vi "IntakeStateMachine.vi"(6 "IntakeCurrent":dbl, 8 "SlowButton":bool, 9 "FastButton":bool, 10 "Joystick":dbl(slide) scale=-1.0..1.0, 11 "Cluster":T1={"OutakeSpeed"=0.4, "OutakeSpeed Fast"=1.0, "Intake Sens"=1.2, "OutakeSens"=0.7} {"OutakeSpeed Fast" format="%#_13g"; "OutakeSpeed" format="%#_13g"}) -> (2 "Left Intake":dbl format="%#_13g", 3 "Right Intake":dbl)   [LabVIEW 2017]
uses:
  Implementation/IntakeStates.ctl
panel:
  out "Waveform Chart":dbl(graph)
  in  "DislodgingLeftSpeed":dbl=-0.2 format="%#_13g"
  in  "DislodgingRightSpeed":dbl=-1.0 format="%#_13g"
  in  "Time Limit":u32=300
  in  "Max Curretnt":dbl=55.0
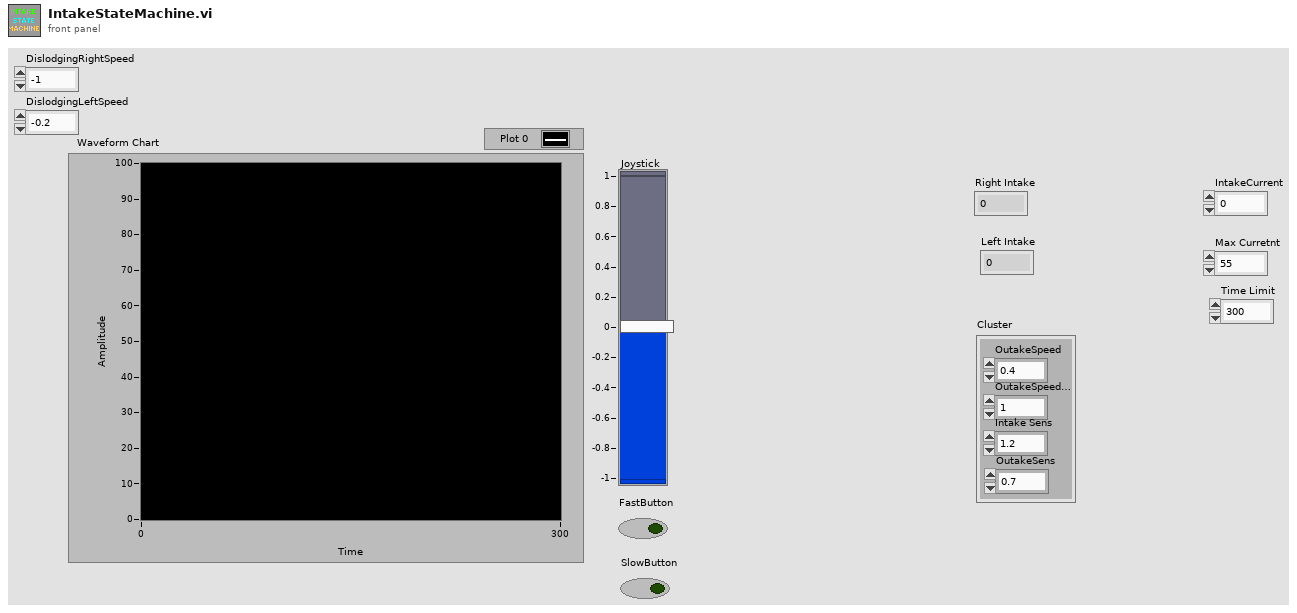
[diagram p1: front panel]
types:
  T1 = cluster{"OutakeSpeed":dbl, "OutakeSpeed Fast":dbl, "Intake Sens":dbl, "OutakeSens":dbl}
  T2 = typedef "IntakeStates.ctl" = enum16{"Intake Manual", "Outtake Manual", "Fast Auto Outake", "Slow Auto Outake", "Dislodging"}
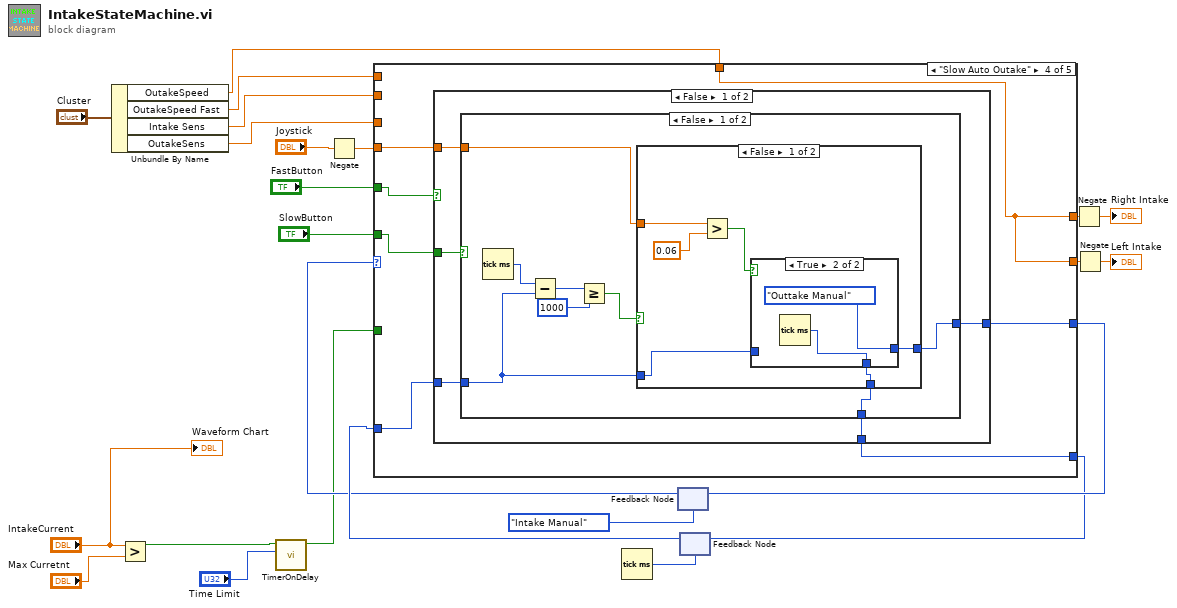
[diagram p0: block diagram]
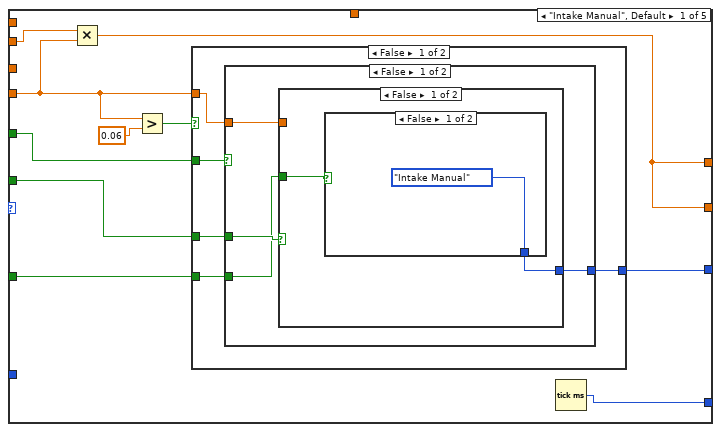
[diagram p2: hidden frame]
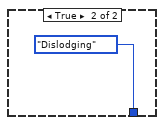
[diagram p3: hidden frame]
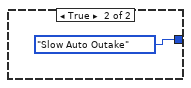
[diagram p4: hidden frame]
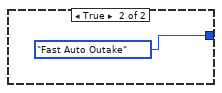
[diagram p5: hidden frame]
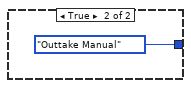
[diagram p6: hidden frame]
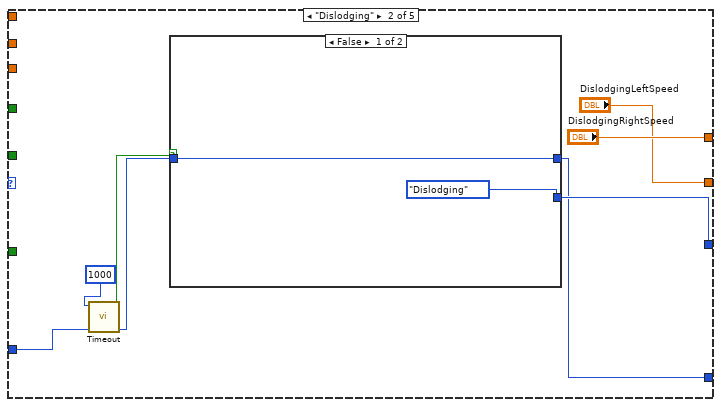
[diagram p7: hidden frame]
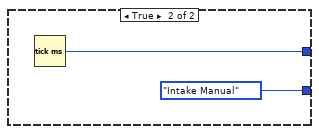
[diagram p8: hidden frame]
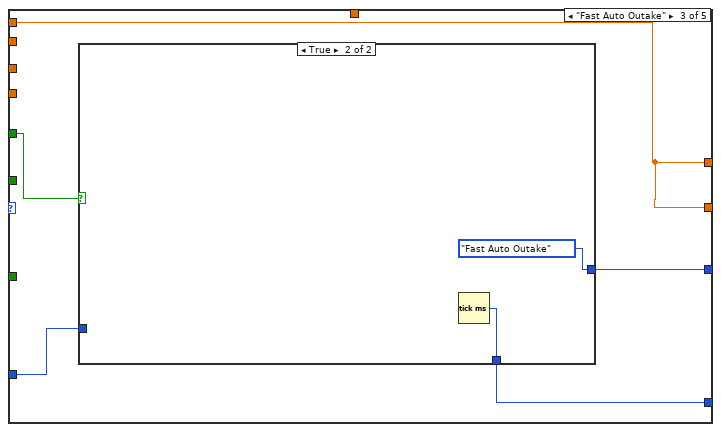
[diagram p9: hidden frame]
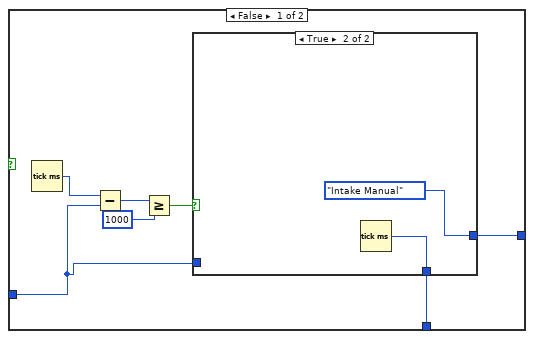
[diagram p10: hidden frame]
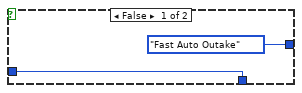
[diagram p11: hidden frame]
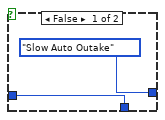
[diagram p12: hidden frame]
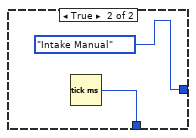
[diagram p13: hidden frame]
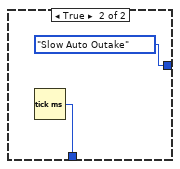
[diagram p14: hidden frame]
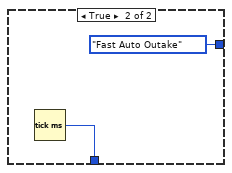
[diagram p15: hidden frame]
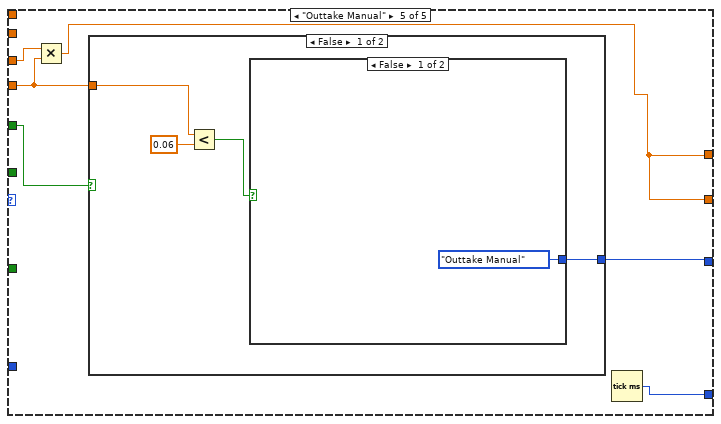
[diagram p16: hidden frame]
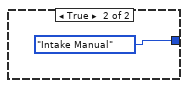
[diagram p17: hidden frame]
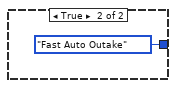
[diagram p18: hidden frame]
diagram:
  n1 = Unbundle By Name("Cluster") -> ("OutakeSpeed"=w14:dbl, "OutakeSpeed Fast"=w15:dbl, "Intake Sens"=w12:dbl, "OutakeSens"=w13:dbl)
  n2 = Greater?(x="IntakeCurrent", y="Max Curretnt") -> (0:w4:bool)
  n3 = call "TimerOnDelay.vi"("Time Limit"="Time Limit", "Input"=w4) -> ("Output"=w2:bool)  [unwired: 9 in]
  n4 = Negate(x="Joystick") -> (-x=w9:dbl)
  n5 = Tick Count (ms)() -> (millisecond timer value=w20:u32)
  n6 = feedback #1(IntakeStates."Intake Manual" ("States")) -> (w11:T2)
  n7 = feedback #2(w20) -> (w19:u32)
  n8 = case shown="\"Slow Auto Outake\"" w11 {
    tunnel: [w26 "DislodgingRightSpeed" w63 w81 w117] -> w17
    tunnel: [w32 w53 w65 w86 w120] -> w23
    tunnel: w9 -> [w28 _ _ w82 w118]
    tunnel: "FastButton" -> [w31 _ w67 w83 w121]
    tunnel: "SlowButton" -> [w30 _ _ w84 _]
    tunnel: w14 -> [_ _ _ w81 _]
    tunnel: w19 -> [_ w56 w64 w85 _]
    tunnel: [w29 w52 w66 w87 w122] -> w18
    tunnel: w15 -> [_ _ w63 _ _]
    tunnel: w13 -> [_ _ _ _ w119]
    tunnel: w12 -> [w27 _ _ _ _]
    tunnel: [w26 "DislodgingLeftSpeed" w63 w81 w117] -> w6
    tunnel: w2 -> [w25 _ _ _ _]
    frame "Intake Manual", Default {
      n9 = Multiply(x=w27, y=w28) -> (x*y=w26:dbl)
      n10 = Greater?(x=w28, y=0.06) -> (0:w33:bool)
      n11 = case shown="False" w33 {
        tunnel: [w38 IntakeStates."Outtake Manual" ("States")] -> w32
        tunnel: w28 -> [w36 _]
        tunnel: w31 -> [w39 _]
        tunnel: w30 -> [w37 _]
        tunnel: w25 -> [w35 _]
        frame False {
          n12 = case shown="False" w39 {
            tunnel: [w42 IntakeStates."Fast Auto Outake" ("States")] -> w38
            tunnel: w37 -> [w43 _]
            tunnel: w36 -> [w41 _]
            tunnel: w35 -> [w40 _]
            frame False {
              n13 = case shown="False" w43 {
                tunnel: [w44 IntakeStates."Slow Auto Outake" ("States")] -> w42
                tunnel: w41 -> [_ _]
                tunnel: w40 -> [w45 _]
                frame False {
                  n14 = case shown="False" w45 {
                    tunnel: [IntakeStates."Intake Manual" ("States") IntakeStates."Dislodging" ("States")] -> w44
                    frame False {
                    }
                    frame True {
                    }
                  }
                }
                frame True {
                }
              }
            }
            frame True {
            }
          }
        }
        frame True {
        }
      }
      n15 = Tick Count (ms)() -> (millisecond timer value=w29:u32)
    }
    frame "Dislodging" {
      n16 = call "Timeout.vi"("Start Time In"=w56, "Time Limit (ms)"=u32 1000) -> ("Start Time Out"=w51:u32, "Timeout"=w54:bool)  [unwired: 8 in]
      n17 = case shown="False" w54 {
        tunnel: [IntakeStates."Dislodging" ("States") IntakeStates."Intake Manual" ("States")] -> w53
        tunnel: [w59 w61] -> w52
        tunnel: w51 -> [w59 _]
        frame False {
        }
        frame True {
          n18 = Tick Count (ms)() -> (millisecond timer value=w61:u32)
        }
      }
    }
    frame "Fast Auto Outake" {
      n19 = case shown="True" w67 {
        tunnel: [w69 w80] -> w66
        tunnel: [w70 IntakeStates."Fast Auto Outake" ("States")] -> w65
        tunnel: w64 -> [w68 _]
        frame False {
          n20 = Tick Count (ms)() -> (millisecond timer value=w74:u32)
          n21 = Subtract(x=w74, y=w68) -> (x-y=w73:u32)
          n22 = Greater Or Equal?(x=w73, y=u32 1000) -> (x >= y?=w71:bool)
          n23 = case shown="True" w71 {
            tunnel: [IntakeStates."Fast Auto Outake" ("States") IntakeStates."Intake Manual" ("States")] -> w70
            tunnel: [w75 w77] -> w69
            tunnel: w68 -> [w75 _]
            frame False {
            }
            frame True {
              n24 = Tick Count (ms)() -> (millisecond timer value=w77:u32)
            }
          }
        }
        frame True {
          n25 = Tick Count (ms)() -> (millisecond timer value=w80:u32)
        }
      }
    }
    frame "Slow Auto Outake" {
      n26 = case shown="False" w83 {
        tunnel: [w92 w115] -> w87
        tunnel: [w91 IntakeStates."Fast Auto Outake" ("States")] -> w86
        tunnel: w85 -> [w90 _]
        tunnel: w84 -> [w89 _]
        tunnel: w82 -> [w88 _]
        frame False {
          n27 = case shown="False" w89 {
            tunnel: [w95 w114] -> w92
            tunnel: [w96 IntakeStates."Slow Auto Outake" ("States")] -> w91
            tunnel: w90 -> [w94 _]
            tunnel: w88 -> [w93 _]
            frame False {
              n28 = Tick Count (ms)() -> (millisecond timer value=w100:u32)
              n29 = Subtract(x=w100, y=w94) -> (x-y=w99:u32)
              n30 = Greater Or Equal?(x=w99, y=u32 1000) -> (x >= y?=w97:bool)
              n31 = case shown="False" w97 {
                tunnel: [w106 IntakeStates."Intake Manual" ("States")] -> w96
                tunnel: [w101 w111] -> w95
                tunnel: w94 -> [w103 _]
                tunnel: w93 -> [w104 _]
                frame False {
                  n32 = Greater?(x=w104, y=0.06) -> (0:w102:bool)
                  n33 = case shown="True" w102 {
                    tunnel: [IntakeStates."Slow Auto Outake" ("States") IntakeStates."Outtake Manual" ("States")] -> w106
                    tunnel: w103 -> [w107 _]
                    tunnel: [w107 w109] -> w101
                    frame False {
                    }
                    frame True {
                      n34 = Tick Count (ms)() -> (millisecond timer value=w109:u32)
                    }
                  }
                }
                frame True {
                  n35 = Tick Count (ms)() -> (millisecond timer value=w111:u32)
                }
              }
            }
            frame True {
              n36 = Tick Count (ms)() -> (millisecond timer value=w114:u32)
            }
          }
        }
        frame True {
          n37 = Tick Count (ms)() -> (millisecond timer value=w115:u32)
        }
      }
    }
    frame "Outtake Manual" {
      n38 = Multiply(x=w119, y=w118) -> (x*y=w117:dbl)
      n39 = case shown="False" w121 {
        tunnel: [w124 IntakeStates."Fast Auto Outake" ("States")] -> w120
        tunnel: w118 -> [w126 _]
        frame False {
          n40 = Less?(x=w126, y=0.06) -> (x < y?=w123:bool)
          n41 = case shown="False" w123 {
            tunnel: [IntakeStates."Outtake Manual" ("States") IntakeStates."Intake Manual" ("States")] -> w124
            frame False {
            }
            frame True {
            }
          }
        }
        frame True {
        }
      }
      n42 = Tick Count (ms)() -> (millisecond timer value=w122:u32)
    }
  }
  n43 = feedback-in #1(w23) -> ()
  n44 = feedback-in #2(w18) -> ()
  n45 = Negate(x=w17) -> (-x=→"Right Intake":dbl)
  n46 = Negate(x=w6) -> (-x=→"Left Intake":dbl)
  "Waveform Chart" <- "IntakeCurrent"
